vi "Lex Value.vi"(8 "error in (no error)":errorcluster, 11 "JSON Lexer in":refnum<class "JSON Lexer.lvclass">) -> (0 "error out":errorcluster, 1 "EOF":bool, 2 "Next State":T1=enum."Value", 3 "JSON Lexer out":refnum<class "JSON Lexer.lvclass">)   [LabVIEW 2019, in "JKI JSON Serialization.lvlib" / "JSON Lexer.lvclass"]
doc: "JKI JSON 1.1.10.37\nTomi Maila - JKI\nCopyright (c) 2017, JKI"
uses:
  JSON Lexer.lvclass
  JSON Lexer States.ctl
  JSON Lexer.lvclass/JSON Lexer.ctl
  Unicode/UTF-8 String/UTF-8 String.lvclass/UTF-8 String.ctl
  JSON Token Type.ctl
  Unicode/UTF-8 String/Index Rune as UTF-8 Substring.vi
  Ignore.vi
  Unicode/UTF-8 String/Next Rune As UTF-8 Substring.vi
  Unicode/UTF-8 String/Bytes In Rune.vi
  <vilib>/Utility/error.llb/Error Cluster From Error Code.vi
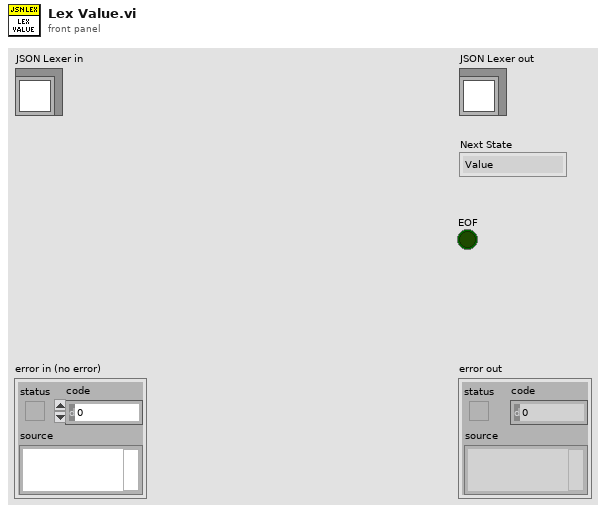
[diagram p1: front panel]
types:
  T1 = typedef "JKI JSON Serialization.lvlib/JSON Lexer.lvclass/JSON Lexer States.ctl" = enum16{"Undefined", "Value", "String", "Numeric", "Number", "Symbol", "Symbolic Number"}
  T2 = typedef "JKI JSON Serialization.lvlib/JSON Lexer.lvclass/JSON Token Type.ctl" = enum32{"unknown", "comma", "end-label", "begin-object", "end-object", "begin-array", "end-array", "quoted-string", "boolean", "exponential-number", "decimal-number", "integer-number", "special-number", "null", "symbol", "whitespace", "EOF"}
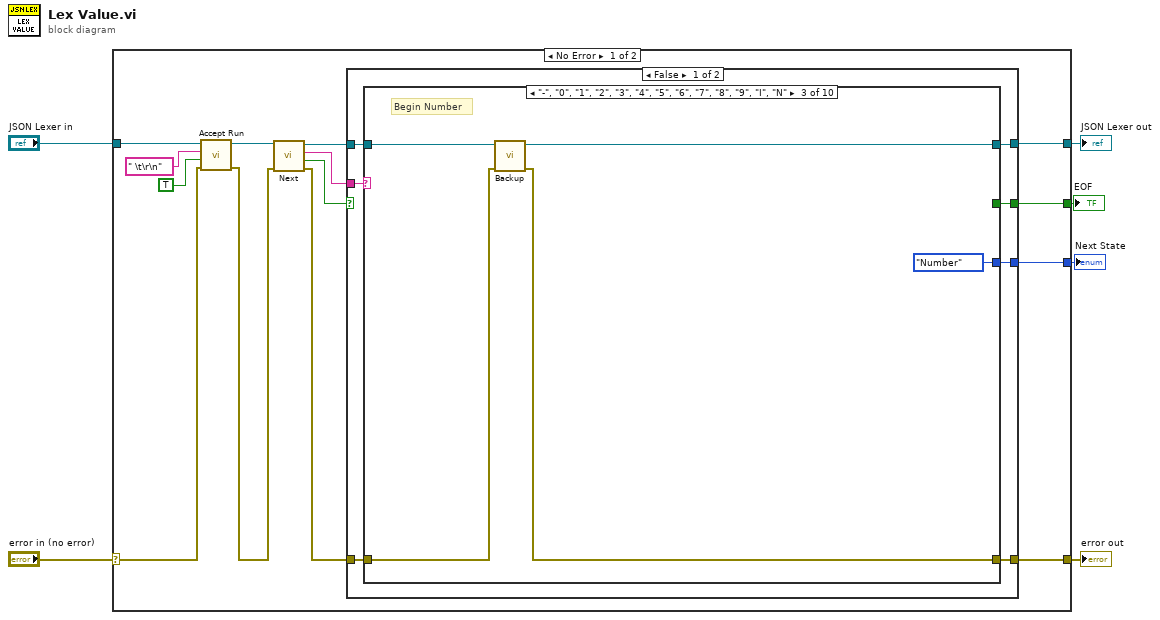
[diagram p0: block diagram]
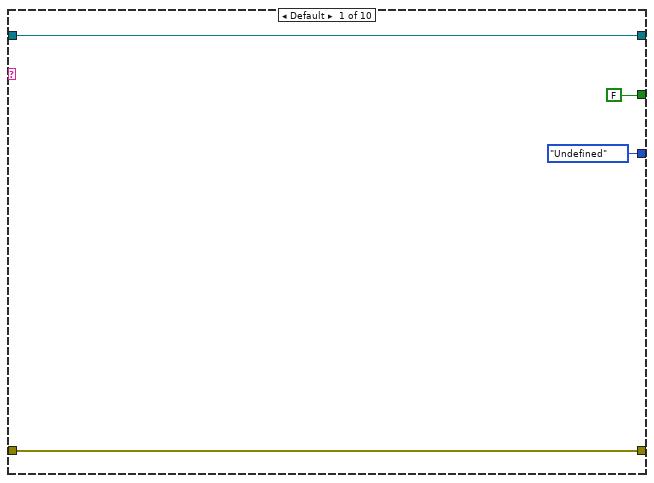
[diagram p2: hidden frame]
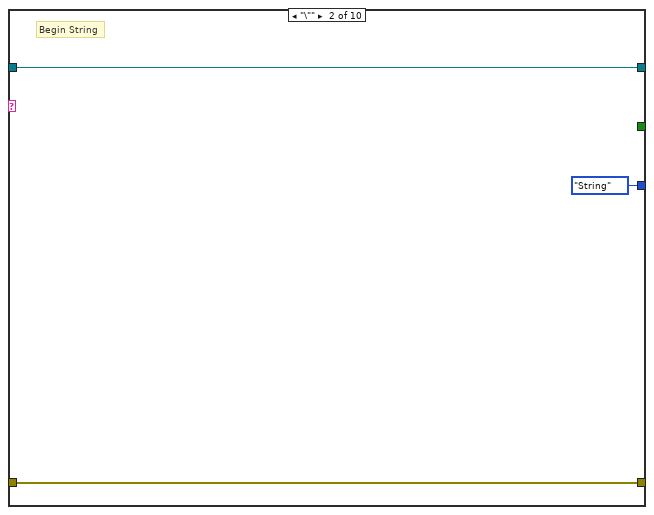
[diagram p3: hidden frame]
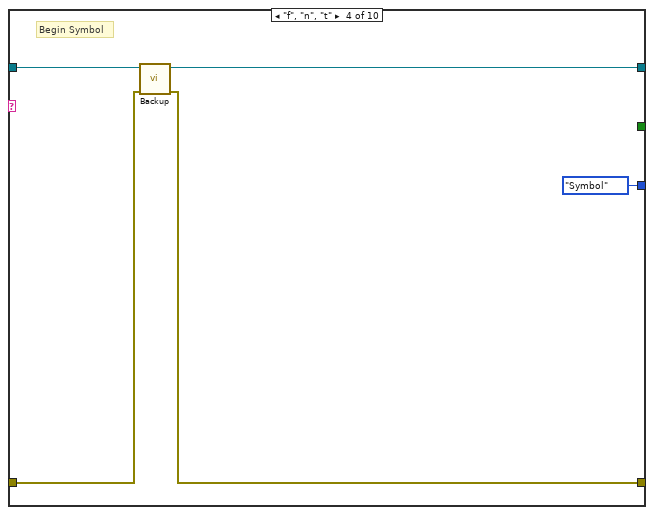
[diagram p4: hidden frame]
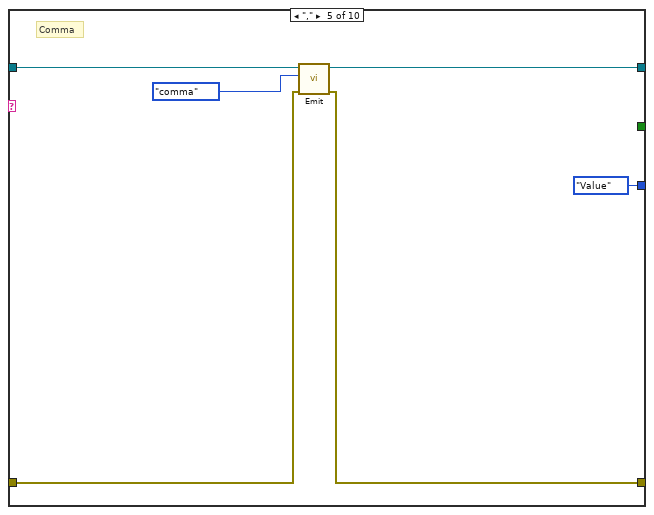
[diagram p5: hidden frame]
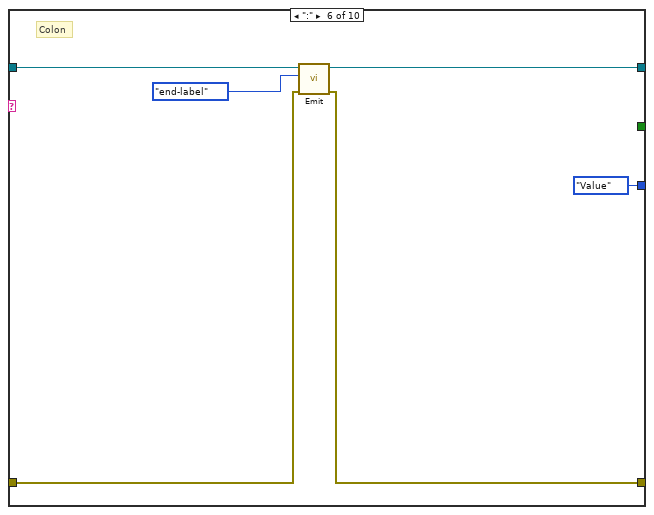
[diagram p6: hidden frame]
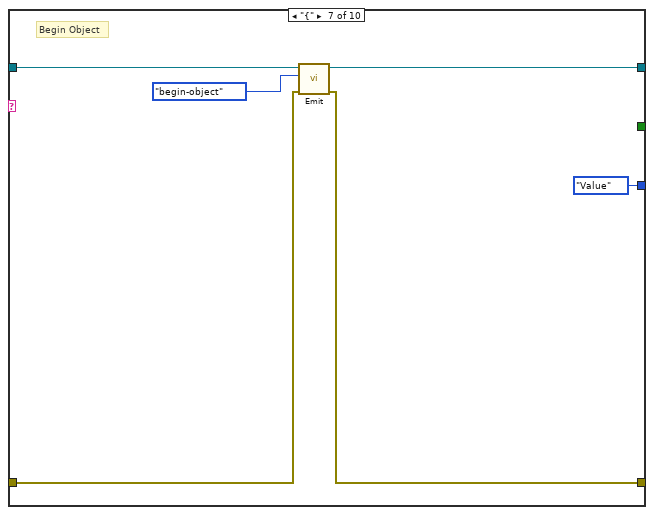
[diagram p7: hidden frame]
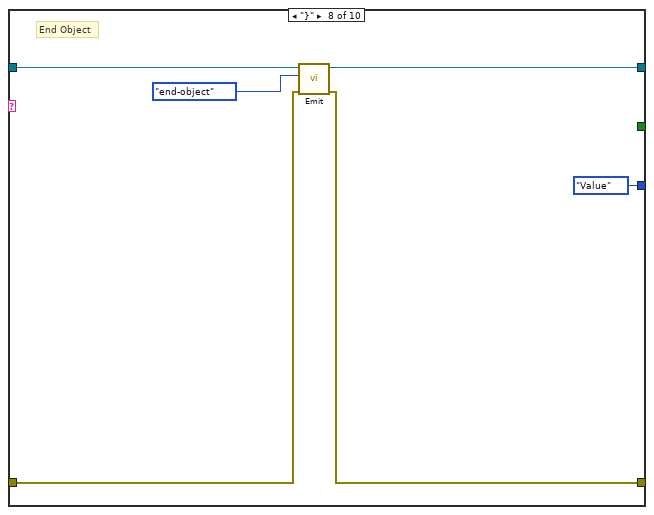
[diagram p8: hidden frame]
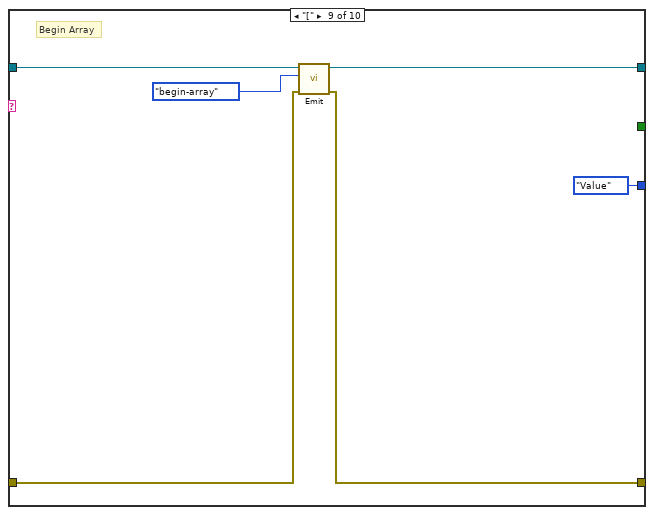
[diagram p9: hidden frame]
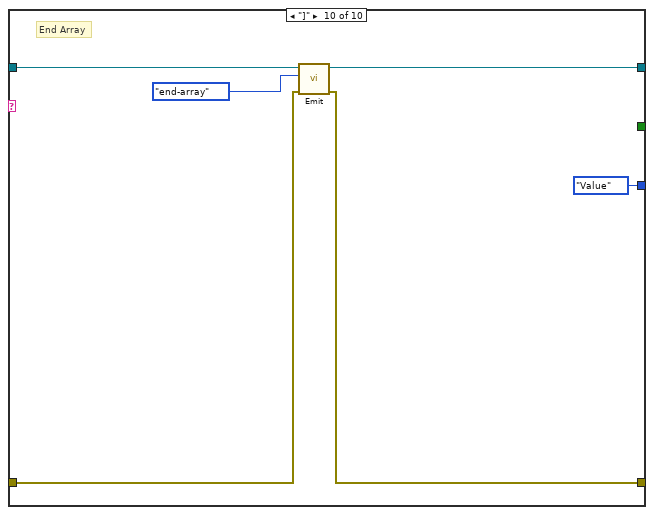
[diagram p10: hidden frame]
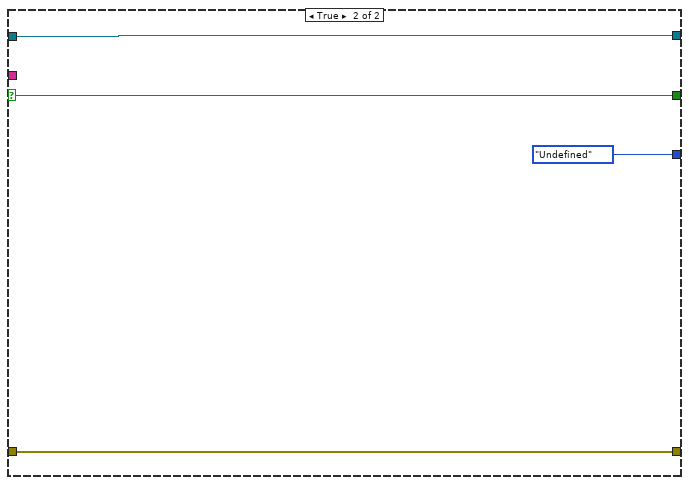
[diagram p11: hidden frame]
diagram:
  n1 = case shown="No Error" "error in (no error)" {
    selector: "error in (no error)" -> [w10 w86]
    tunnel: [w16 w86] -> w5
    tunnel: [w15 w85] -> w3
    tunnel: "JSON Lexer in" -> [w12 w85]
    tunnel: [w14 _] -> w2
    tunnel: [w13 _] -> w1
    frame No Error {
      n2 = call "Accept Run.vi"("error in (no error)"=w10, "Ignore"=TRUE, "Accepted Runes"=" \t\r\n", "JSON Lexer in"=w12) -> ("error out"=w9:errorcluster, "JSON Lexer out"=w11:refnum<class "JSON Lexer.lvclass">)  [unwired: 6 in]
      n3 = call "Next.vi"("error in (no error)"=w9, "JSON Lexer in"=w11) -> ("error out"=w17:errorcluster, "EOF"=w20:bool, "Rune"=w19:string, "JSON Lexer out"=w18:refnum<class "JSON Lexer.lvclass">)  [unwired: 6 in]
      n4 = case shown="False" w20 {
        selector: w20 -> [_ w82]
        tunnel: w19 -> [w25 _]
        tunnel: w18 -> [w27 w84]
        tunnel: w17 -> [w24 w83]
        tunnel: [w23 w83] -> w16
        tunnel: [w26 w84] -> w15
        tunnel: [w22 w82] -> w14
        tunnel: [w21 JSON_Lexer_States."Undefined" ("Next State")] -> w13
        frame False {
          n5 = case shown="\"-\", \"0\", \"1\", \"2\", \"3\", \"4\", \"5\", \"6\", \"7\", \"8\", \"9\", \"I\", \"N\"" w25 {
            tunnel: w27 -> [w31 w34 w38 w43 w49 w55 w61 w67 w73 w79]
            tunnel: [w31 w34 w37 w42 w48 w54 w60 w66 w72 w78] -> w26
            tunnel: w24 -> [w30 w33 w36 w41 w46 w52 w58 w64 w70 w76]
            tunnel: [w30 w33 w35 w40 w45 w51 w57 w63 w69 w75] -> w23
            tunnel: [FALSE _ _ _ _ _ _ _ _ _] -> w22
            tunnel: [JSON_Lexer_States."Undefined" ("Next State") JSON_Lexer_States."String" ("Next State") JSON_Lexer_States."Number" ("Next State") JSON_Lexer_States."Symbol" ("Next State") JSON_Lexer_States."Value" ("Next State") JSON_Lexer_States."Value" ("Next State") JSON_Lexer_States."Value" ("Next State") JSON_Lexer_States."Value" ("Next State") JSON_Lexer_States."Value" ("Next State") JSON_Lexer_States."Value" ("Next State")] -> w21
            frame Default {
            }
            frame "\"" {
              # "Begin String"
            }
            frame "-", "0", "1", "2", "3", "4", "5", "6", "7", "8", "9", "I", "N" {
              # "Begin Number"
              n6 = call "Backup.vi"("error in (no error)"=w36, "JSON Lexer in"=w38) -> ("error out"=w35:errorcluster, "JSON Lexer out"=w37:refnum<class "JSON Lexer.lvclass">)  [unwired: 8 in]
            }
            frame "f", "n", "t" {
              # "Begin Symbol"
              n7 = call "Backup.vi"("error in (no error)"=w41, "JSON Lexer in"=w43) -> ("error out"=w40:errorcluster, "JSON Lexer out"=w42:refnum<class "JSON Lexer.lvclass">)  [unwired: 8 in]
            }
            frame "," {
              # "Comma"
              n8 = call "Emit.vi"("error in (no error)"=w46, "JSON Token Type"=JSON_Token_Type."comma", "JSON Lexer in"=w49) -> ("error out"=w45:errorcluster, "JSON Lexer out"=w48:refnum<class "JSON Lexer.lvclass">)  [unwired: 7 in]
            }
            frame ":" {
              # "Colon"
              n9 = call "Emit.vi"("error in (no error)"=w52, "JSON Token Type"=JSON_Token_Type."end-label", "JSON Lexer in"=w55) -> ("error out"=w51:errorcluster, "JSON Lexer out"=w54:refnum<class "JSON Lexer.lvclass">)  [unwired: 7 in]
            }
            frame "{" {
              # "Begin Object"
              n10 = call "Emit.vi"("error in (no error)"=w58, "JSON Token Type"=JSON_Token_Type."begin-object", "JSON Lexer in"=w61) -> ("error out"=w57:errorcluster, "JSON Lexer out"=w60:refnum<class "JSON Lexer.lvclass">)  [unwired: 7 in]
            }
            frame "}" {
              # "End Object"
              n11 = call "Emit.vi"("error in (no error)"=w64, "JSON Token Type"=JSON_Token_Type."end-object", "JSON Lexer in"=w67) -> ("error out"=w63:errorcluster, "JSON Lexer out"=w66:refnum<class "JSON Lexer.lvclass">)  [unwired: 7 in]
            }
            frame "[" {
              # "Begin Array"
              n12 = call "Emit.vi"("error in (no error)"=w70, "JSON Token Type"=JSON_Token_Type."begin-array", "JSON Lexer in"=w73) -> ("error out"=w69:errorcluster, "JSON Lexer out"=w72:refnum<class "JSON Lexer.lvclass">)  [unwired: 7 in]
            }
            frame "]" {
              # "End Array"
              n13 = call "Emit.vi"("error in (no error)"=w76, "JSON Token Type"=JSON_Token_Type."end-array", "JSON Lexer in"=w79) -> ("error out"=w75:errorcluster, "JSON Lexer out"=w78:refnum<class "JSON Lexer.lvclass">)  [unwired: 7 in]
            }
          }
        }
        frame True {
        }
      }
    }
    frame Error {
    }
  }
  "error out" <- w5
  "JSON Lexer out" <- w3
  "Next State" <- w1
  "EOF" <- w2
